vi "Quasi Random.vi"   [LabVIEW 2017, in "NI_AAL_SignalGeneration.lvlib"]
doc: "Generates quasi-random Halton or Richtmeyer sequences, which are low-discrepancy number sequences."
uses:
  <vilib>/Analysis/NI_AAL_SignalGeneration.lvlib
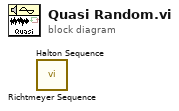
[diagram p0: block diagram]
diagram:
  n1 = call <vilib>:"Richtmeyer Sequence.vi"() -> ()  [unwired: 10 in, 2 out]
  n2 = call <vilib>:"Halton Sequence.vi"() -> ()  [unwired: 10 in, 2 out]
